vi "Parse Event Name from ref.vi"(10 "Boolean Run Request VI":refnum<vi>, 11 "VI in":refnum<vi>) -> ()   [LabVIEW 2020, in "DQMH_API.lvlib"]
uses:
  DQMH_API.lvlib
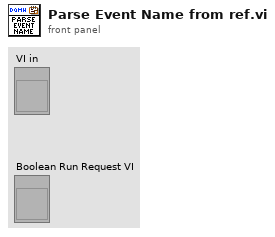
[diagram p1: front panel]
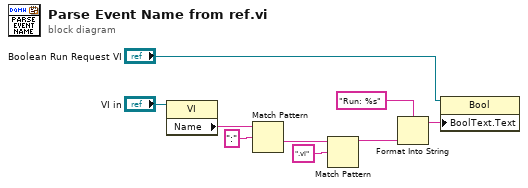
[diagram p0: block diagram]
diagram:
  n1 = property class="VI"(reference="VI in") -> ("Name"=w5:string)  [unwired: 1 in, 2 out]
  n2 = Match Pattern(string=w5, regular expression=":") -> (after substring=w3:string)  [unwired: 1 in, 3 out]
  n3 = Match Pattern(string=w3, regular expression=".vi") -> (before substring=w1:string)  [unwired: 1 in, 3 out]
  n4 = Format Into String(format string="Run: %s", w1) -> (resulting string=w7:string)  [unwired: 2 in, 1 out]
  n5 = property on="Property Node" class="Bool"(reference="Boolean Run Request VI", "BoolText.Text"=w7) -> ()  [unwired: 1 in, 2 out]
